vi "ARRAY2.vi"(10 "row to sort":dbl, 11 "Array in":dbl[][](array[numeric])) -> (1 "output array":dbl[][](array[numeric]), 2 "sorted array":dbl[](array[numeric]), 3 "Array out":dbl[][](array[numeric]))   [LabVIEW 2018]
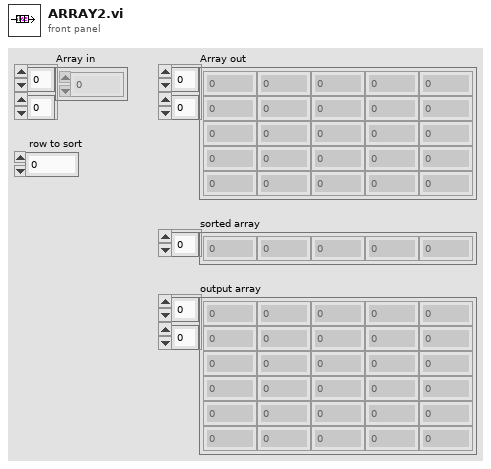
[diagram p1: front panel]
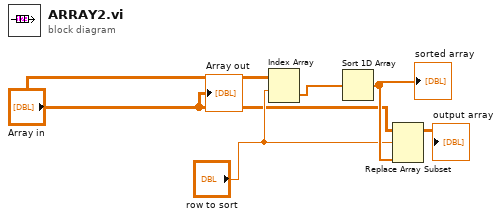
[diagram p0: block diagram]
diagram:
  n1 = Index Array(array="Array in", index (row)="row to sort") -> (element=w1:dbl[])  [unwired: 1 in]
  n2 = Sort 1D Array(array=w1) -> (sorted array=w5:dbl[])
  "sorted array" <- w5
  n3 = Replace Array Subset(array="Array in", new element=w5, index (row)="row to sort") -> (→"output array":dbl[][])  [unwired: 1 in]
  "Array out" <- "Array in"
